vi "GOLPI full test - part structure.vi"(8 "error in":errorcluster, 11 "GOLPI ref. in":T1={"pipe handle"={"lv_proc.dll file path"=path "", "process instance handle"=[], "debug mode"=FALSE, "debug data"=[]}, "fast read timeout [ms]"=500, "fast read settle time [ms]"=10, "fast read to multiple [ms]"=1, "max elements per input line"=100, "slow read timeout [ms]"=5000, "stdin double format specifier"="", "max elements per stdout output column"=100, "console mode bitstream"=FALSE, "bitstream first read timeout [ms]"=1000, "bitstream read timeout [ms]"=50, "struct transfer possible"=FALSE}) -> (0 "error out":errorcluster, 2 "match":bool, 3 "GOLPI ref. out":T1={"pipe handle"={"lv_proc.dll file path"=path "", "process instance handle"=[], "debug mode"=FALSE, "debug data"=[]}, "fast read timeout [ms]"=500, "fast read settle time [ms]"=10, "fast read to multiple [ms]"=1, "max elements per input line"=100, "slow read timeout [ms]"=5000, "stdin double format specifier"="%_16e", "max elements per stdout output column"=100, "console mode bitstream"=FALSE, "bitstream first read timeout [ms]"=1000, "bitstream read timeout [ms]"=50, "struct transfer possible"=FALSE})   [LabVIEW 2013, in "GOLPI library.lvlib"]
uses:
  GOLPI library.lvlib
  Public/GOLPI reference Type Def.ctl
  LV Process source distribution/Pipe Handle.ctl
  LV Process source distribution/LV Process library.lvlib
panel:
  in  "struct":T3
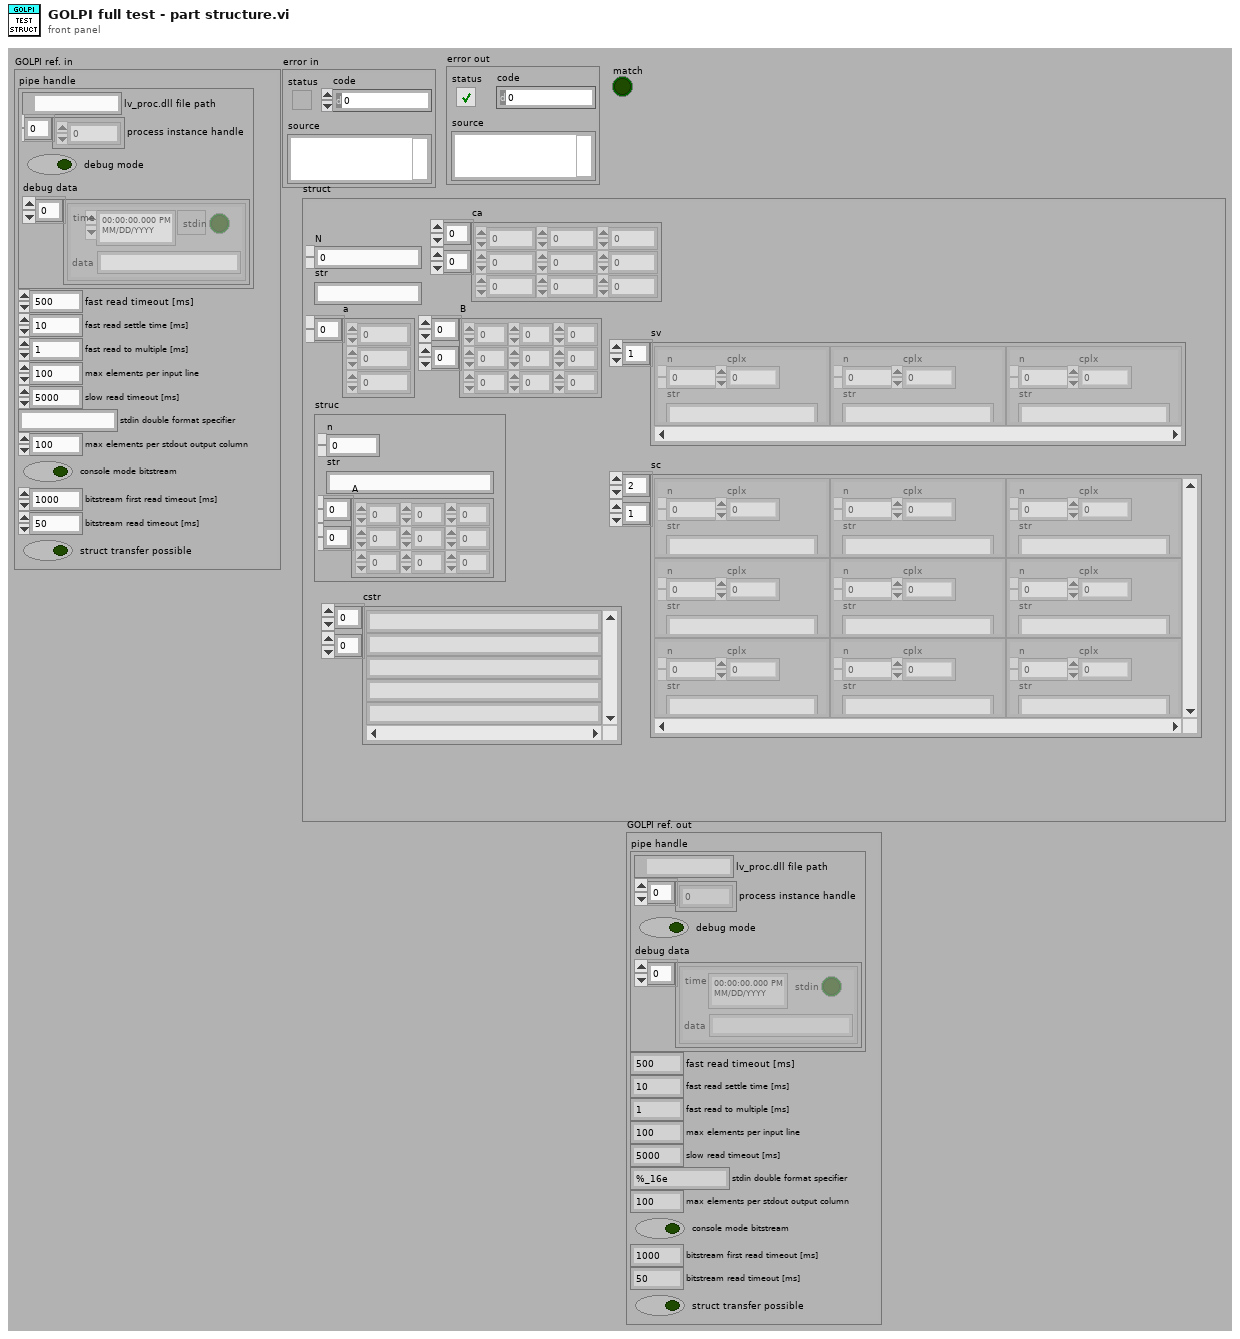
[diagram p1: front panel]
types:
  T1 = typedef "GOLPI library.lvlib/GOLPI reference Type Def.ctl" = cluster{"pipe handle":T2, "fast read timeout [ms]":u32, "fast read settle time [ms]":u32, "fast read to multiple [ms]":u32, "max elements per input line":u32, "slow read timeout [ms]":u32, "stdin double format specifier":string, "max elements per stdout output column":u32, "console mode bitstream":bool, "bitstream first read timeout [ms]":u32, "bitstream read timeout [ms]":u32, "struct transfer possible":bool}
  T2 = typedef "LV Process library.lvlib/Pipe Handle.ctl" = cluster{"lv_proc.dll file path":path, "process instance handle":u32[], "debug mode":bool, "debug data":cluster{"time":timestamp, "stdin":bool, "data":string}[]}
  T3 = cluster{"N":dbl, "str":string, "a":i32[], "struc":cluster{"n":dbl, "str":string, "A":dbl[][]}, "B":dbl[][], "ca":cdb[][], "sv":cluster{"n":dbl, "str":string, "cplx":cdb}[], "sc":cluster{"n":dbl, "str":string, "cplx":cdb}[][], "cstr":string[][]}
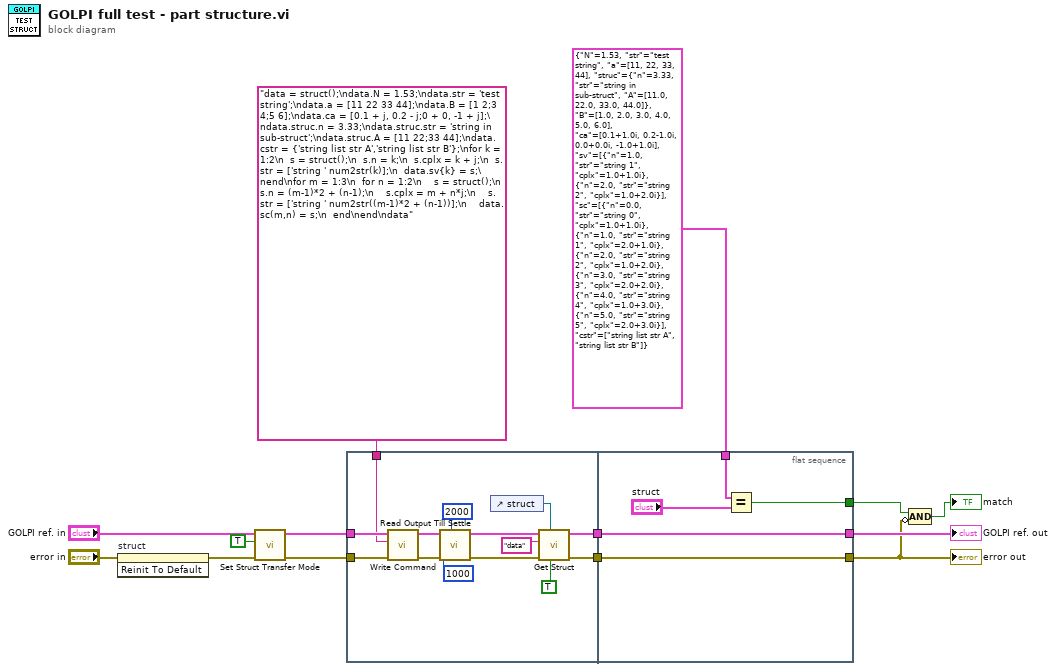
[diagram p0: block diagram]
diagram:
  n1 = invoke on="struct" class="Clust (strict)" method="Reinit To Default"(error in="error in") -> (error out=w1:errorcluster)  [unwired: 2 in, 2 out]
  n2 = call "Set Struct Transfer Mode.vi"("error in"=w1, "Allow struct tranfer (False)"=TRUE, "GOLPI ref. in"="GOLPI ref. in") -> ("error out"=w12:errorcluster, "GOLPI ref. out"=w11:T1)  [unwired: 6 in, 1 out]
  n3 = flat-sequence {
    tunnel: w12 -> [w26]
    tunnel: w11 -> [w24]
    tunnel: "data = struct();\ndata.N = 1.53;\ndata.str = 'test string';\ndata.a = [11 22 33 44];\ndata.B = [1 2;3 4;5 6];\ndata.ca = [0.1 + j, 0.2 - j;0 + 0, -1 + j];\ndata.struc.n = 3.33;\ndata.struc.str = 'string in sub-struct';\ndata.struc.A = [11 22;33 44];\ndata.cstr = {'string list str A','string list str B'};\nfor k = 1:2\n  s = struct();\n  s.n = k;\n  s.cplx = k + j;\n  s.str = ['string ' num2str(k)];\n  data.sv{k} = s;\nend\nfor m = 1:3\n  for n = 1:2\n    s = struct();\n    s.n = (m-1)*2 + (n-1);\n    s.cplx = m + n*j;\n    s.str = ['string ' num2str((m-1)*2 + (n-1))];\n    data.sc(m,n) = s;\n  end\nend\ndata" -> [w23]
    tunnel: [w22] -> w9
    tunnel: [w21] -> w8
    tunnel: w9 -> [w33]
    tunnel: w8 -> [w32]
    tunnel: [w33] -> w5
    tunnel: [w32] -> w7
    tunnel: T3 {"N"=1.53, "str"="test string", "a"=[11, 22, 33, 44], "struc"={"n"=3.33, "str"="string in sub-struct", "A"=[[11.0, 22.0], [33.0, 44.0]]}, "B"=[[1.0, 2.0], [3.0, 4.0], [5.0, 6.0]], "ca"=[[0.1+1.0i, 0.2-1.0i], [0.0+0.0i, -1.0+1.0i]], "sv"=[{"n"=1.0, "str"="string 1", "cplx"=1.0+1.0i}, {"n"=2.0, "str"="string 2", "cplx"=1.0+2.0i}], "sc"=[[{"n"=0.0, "str"="string 0", "cplx"=1.0+1.0i}, {"n"=1.0, "str"="string 1", "cplx"=2.0+1.0i}], [{"n"=2.0, "str"="string 2", "cplx"=1.0+2.0i}, {"n"=3.0, "str"="string 3", "cplx"=2.0+2.0i}], [{"n"=4.0, "str"="string 4", "cplx"=1.0+3.0i}, {"n"=5.0, "str"="string 5", "cplx"=2.0+3.0i}]], "cstr"=[["string list str A", "string list str B"]]} ("struct") -> [w30]
    tunnel: [w29] -> w4
    frame #0 {
      n4 = call "Write Command.vi"("error in"=w26, "command"=w23, "GOLPI ref. in"=w24) -> ("error out"=w20:errorcluster, "GOLPI ref. out"=w19:T1)  [unwired: 7 in]
      n5 = call "Read Output Till Settle.vi"("timeout [ms]"=u32 2000, "error in"=w20, "settled for [ms]"=u32 1000, "GOLPI ref. in"=w19) -> ("error out"=w18:errorcluster, "GOLPI ref. out"=w17:T1)  [unwired: 4 in, 2 out]
      n6 = control-ref of="struct"() -> (w27:refnum<vi>)
      n7 = call "Get Struct.vi"("reinit cluster to default (false)"=TRUE, "cluster ref (empty)"=w27, "error in"=w18, "variable"="data", "GOLPI ref in"=w17) -> ("error out"=w22:errorcluster, "GOLPI ref. out"=w21:T1)  [unwired: 4 in, 1 out]
    }
    frame #1 {
      n8 = Equal?(x=w30, y="struct") -> (x = y?=w29:bool)
    }
  }
  n9 = Compound Arithmetic op=AND(w4, invert w5) -> (→"match":bool)
  "error out" <- w5
  "GOLPI ref. out" <- w7
